vi "G4SubTemplate_Singleton_4x4x4_GetInstance.vi"(8 "Error In":errorcluster, 11 "reference in":refnum<class "G4SubTemplate_Singleton_4x4x4.lvclass"> caption="This control should only be used when\na sub class is inheriting this class") -> (0 "Error Out":errorcluster, 1 "DVRRefOut":refnum<data-value>, 2 "NewObjectCreated":bool, 3 "reference out":refnum<class "G4SubTemplate_Singleton_4x4x4.lvclass">, 5 "ObjectQueueName":string caption="This queue name could be used to destroy\nthe named queue that is used to hold the\nreference in the clean up.")   [LabVIEW 2020, in "G4SubTemplate_Singleton_4x4x4.lvclass"]
uses:
  <resource>/Framework/Providers/Open_GDS/ClassProviders/Provider_EndevoGOOP400/Templates/G4SubTemplate_Singleton_4x4x4/G4SubTemplate_Singleton_4x4x4.lvclass
  <resource>/Framework/Providers/Open_GDS/ClassProviders/Provider_EndevoGOOP400/Templates/G4SubTemplate_Singleton_4x4x4/protected/ObjectAttributes.ctl
  <resource>/Framework/Providers/Open_GDS/ClassProviders/Provider_EndevoGOOP400/Templates/G4SubTemplate_Singleton_4x4x4/G4SubTemplate_Singleton_4x4x4.lvclass/G4SubTemplate_Singleton_4x4x4.ctl
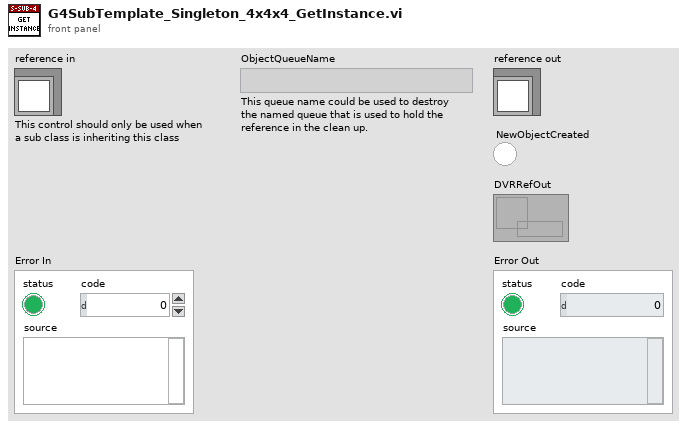
[diagram p1: front panel]
types:
  T1 = enum16{"Create or look up existing", "Look up existing"}
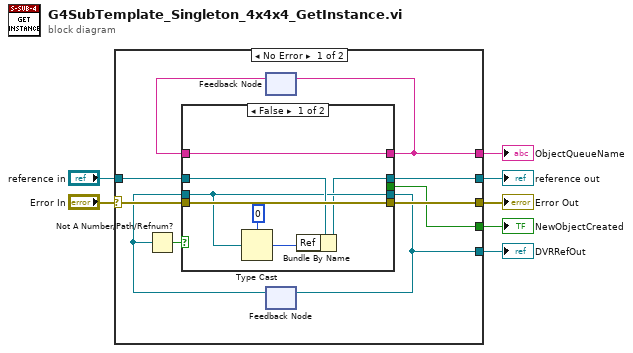
[diagram p0: block diagram]
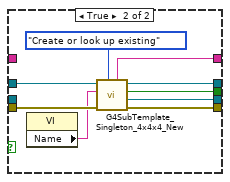
[diagram p2: hidden frame]
diagram:
  n1 = case shown="No Error" "Error In" {
    selector: "Error In" -> [w16 w35]
    tunnel: [w17 w34] -> w7
    tunnel: [w15 w35] -> w5
    tunnel: "reference in" -> [w14 w34]
    tunnel: [w13 _] -> w3
    tunnel: [w12 _] -> w2
    tunnel: [w9 _] -> w1
    frame No Error {
      n2 = feedback #1() -> (w8:string)  [unwired: 1 in]
      n3 = feedback #2() -> (w10:refnum<data-value>)  [unwired: 1 in]
      n4 = Not A Number/Path/Refnum?(number/path/refnum=w10) -> (NaN/Path/Refnum?=w11:bool)
      n5 = case shown="False" w11 {
        tunnel: [w19 w33] -> w17
        tunnel: w16 -> [w24 w32]
        tunnel: [w24 w31] -> w15
        tunnel: w14 -> [w23 w29]
        tunnel: [_ w28] -> w13
        tunnel: [w22 w26] -> w9
        tunnel: [w21 w25] -> w12
        tunnel: w10 -> [w21 _]
        tunnel: w8 -> [w22 _]
        frame False {
          n6 = Type Cast(type=u32 0, x=w21) -> (*(type *) &x=w18:u32)
          n7 = Bundle By Name(cluster=w23, "Ref"=w18) -> (w19:refnum<class "G4SubTemplate_Singleton_4x4x4.lvclass">)
        }
        frame True {
          n8 = property class="VI"() -> ("Name"=w30:string)  [unwired: 2 in, 2 out]
          n9 = call <resource>:"G4SubTemplate_Singleton_4x4x4_New.vi"("CreateMethod(Create or look up existing)"=T1."Create or look up existing", "Error In"=w32, "Object name"=w30, "reference in"=w29) -> ("Error Out"=w31:errorcluster, "DVRRefOut"=w25:refnum<data-value>, "NewObjectCreated"=w28:bool, "reference out"=w33:refnum<class "G4SubTemplate_Singleton_4x4x4.lvclass">, "ObjectQueueName"=w26:string)  [unwired: 3 in]
        }
      }
      n10 = feedback-in #1(w9) -> ()
      n11 = feedback-in #2(w12) -> ()
    }
    frame Error {
    }
  }
  "reference out" <- w7
  "Error Out" <- w5
  "NewObjectCreated" <- w3
  "DVRRefOut" <- w2
  "ObjectQueueName" <- w1
